vi "User form template.vi"   [LabVIEW 2020, in "Panel Form Controller.lvlib"]
uses:
  Panel Form Controller.lvlib
  Database OOP/Table Libraries/Basic Form/Basic Form.lvclass
  Database OOP/Column Libraries/Basic Field Constructors.lvlib
  Open Form Button/Open Form Button.lvclass
  Form Controller/Panel Form Controller.lvclass
  Database OOP/Column Libraries/Basic Field Constructors/Text Field.vi
  C:/Program Files (x86)/National Instruments/LabVIEW 2020/vi.lib/MGI/Panel Manager/Panel Actor/Panel Actor/Panel Actor.lvclass
  C:/Program Files (x86)/National Instruments/LabVIEW 2020/vi.lib/MGI/Monitored Actor/Monitored Actor/Monitored Actor/Monitored Actor.lvclass
  C:/Program Files (x86)/National Instruments/LabVIEW 2020/vi.lib/ActorFramework/Actor/Actor.lvclass
  C:/Users/User/Desktop/Raman Program/Database OOP/source/Forms AF/Forms Controller/Form Controller/Panel Form Controller.lvclass
  C:/Users/User/Desktop/Raman Program/Database OOP/source/Database OOP/Button Libraries/Button/Button Class/Button.lvclass
  C:/Users/User/Desktop/Raman Program/Database OOP/source/Database OOP/Button Libraries/Button Interface Class/Button Interface.lvclass
  C:/Users/User/Desktop/Raman Program/Database OOP/source/Forms AF/Forms Controller/Open Form Button/Open Form Button.lvclass
types:
  T1 = typedef "Panel Form Controller.lvlib/Builder Cluster.ctl" = cluster{"VI Ctrl Array":refnum<vi>[], "Form":refnum<class "Basic Form.lvclass">, "Open Form Button":refnum<class "Open Form Button.lvclass">}
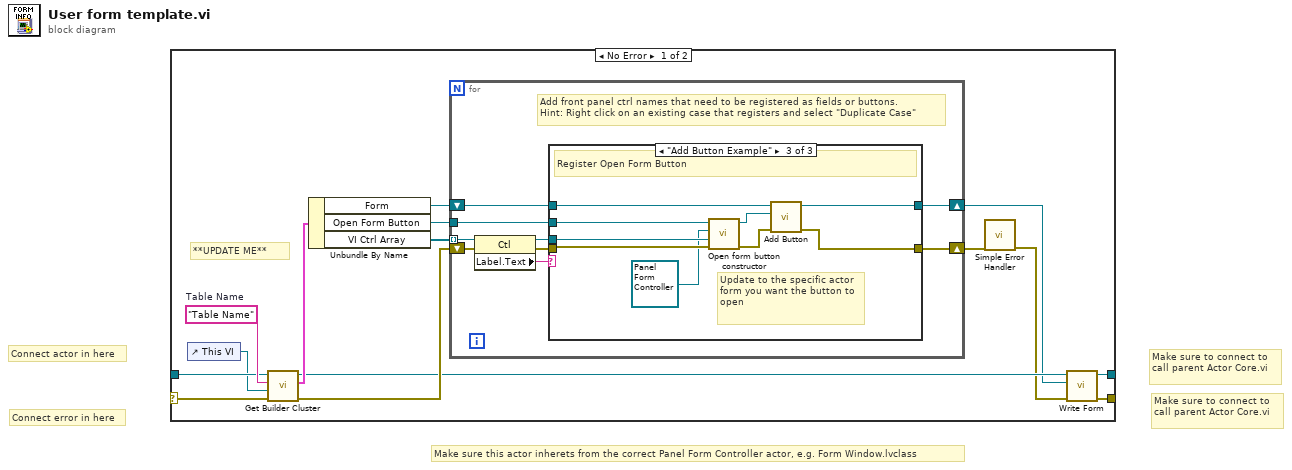
[diagram p0: block diagram]
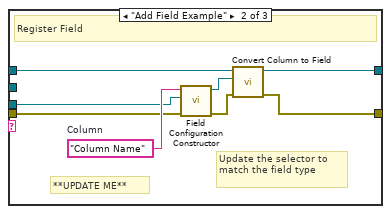
[diagram p3: hidden frame]
diagram:
  # "Make sure to connect to\ncall parent Actor Core.vi"
  # "Make sure to connect to\ncall parent Actor Core.vi"
  # "Make sure this actor inherets from the correct Panel Form Controller actor, e.g. Form Window.lvclass"
  # "Connect error in here"
  # "Connect actor in here"
  n1 = case shown="No Error" {
    selector: _ -> [w12 w45]
    tunnel: _ -> [w2 w44]
    tunnel: [w6 w45] -> _
    tunnel: [w7 w44] -> _
    frame No Error {
      w5 = "Table Name"  # Table Name
      # "**UPDATE ME**"
      n2 = control-ref of="This VI"() -> (w1:refnum<vi>)
      n3 = call "Get Builder Cluster.vi"("error in (no error)"=w12, "VI Refnum"=w1, "Table Name"=w5, "Panel Form Controller in"=w2) -> ("error out"=w14:errorcluster, "Builder Cluster"=w13:T1, "Panel Form Controller out"=w9:refnum<class "Panel Form Controller.lvclass">)  [unwired: 5 in]
      n4 = Unbundle By Name(w13) -> ("Form"=w15:refnum<class "Basic Form.lvclass">, "Open Form Button"=w10:refnum<class "Open Form Button.lvclass">, "VI Ctrl Array"=w11:refnum<vi>[])
      n5 = for {
        tunnel: w11 -> [w24] mode=indexing
        shift-right: [w18] -> w8
        shift-left: w15 -> [w19]
        shift-right: [w16] -> w4
        shift-left: w14 -> [w22]
        tunnel: w10 -> [w17]
        # "Add front panel ctrl names that need to be registered as fields or buttons.\nHint: Right click on an existing case that registers and select \"Duplicate Case\""
        n6 = property class="Ctl"(reference=w24, error in=w22) -> (reference out=w23:refnum<vi>, error out=w21:errorcluster, "Label.Text"=w20:string)
        n7 = case shown="\"Add Button Example\"" w20 {
          tunnel: w23 -> [_ w29 w37]
          tunnel: w19 -> [w26 w34 w43]
          tunnel: [w26 w32 w42] -> w18
          tunnel: [w25 w33 w41] -> w16
          tunnel: w21 -> [w25 w28 w36]
          tunnel: w17 -> [_ _ w38]
          frame "", Default {
            # "Not Registered"
          }
          frame "Add Field Example" {
            w30 = "Column Name"  # Column
            # "Update the selector to match the field type"
            # "**UPDATE ME**"
            # "Register Field"
            n8 = call-poly "Field Configuration Constructor.vi"("error in"=w28, "Ctl Refnum"=w29, "Column Name"=w30) -> ("error out"=w31:errorcluster, "Field Configuration"=w27:refnum<class "Field Configuration.lvclass">)  [unwired: 7 in]
            n9 = call "Convert Column to Field.vi"("error in (no error)"=w31, "Field Configuration"=w27, "Basic Form in"=w34) -> ("error out"=w33:errorcluster, "Basic Form out"=w32:refnum<class "Basic Form.lvclass">)  [unwired: 7 in]
          }
          frame "Add Button Example" {
            # "Update to the specific actor form you want the button to open"
            # "Register Open Form Button"
            n10 = call "Open form button constructor.vi"("error in (no error)"=w36, "Ctl Refnum"=w37, "Panel Form"=refnum<class "Panel Form Controller.lvclass"> refnum ("Panel Form Controller.lvlib:Panel Form Controller.lvclass"), "Open Form Button in"=w38) -> ("error out"=w39:errorcluster, "Open Form Button out"=w40:refnum<class "Open Form Button.lvclass">)  [unwired: 6 in]
            n11 = call "Add Button.vi"("error in (no error)"=w39, "Button"=w40, "Basic Form in"=w43) -> ("error out"=w41:errorcluster, "Basic Form out"=w42:refnum<class "Basic Form.lvclass">)  [unwired: 7 in]
          }
        }
      }
      n12 = call <vilib>:"Simple Error Handler.vi"("error in (no error)"=w4) -> ("error out"=w3:errorcluster)  [unwired: 4 in, 4 out]
      n13 = call "Write Form.vi"("error in (no error)"=w3, "Form.lvlib:Basic Form.lvclass"=w8, "Panel Form Controller in"=w9) -> ("error out"=w6:errorcluster, "Panel Form Controller out"=w7:refnum<class "Panel Form Controller.lvclass">)  [unwired: 7 in]
    }
    frame Error {
    }
  }
